vi "ethernet bc read.vi"(8 "error in":errorcluster, 11 "TCP Network Connection in":refnum<k5>) -> (2 "String":string, 3 "connection ID out":refnum<k5>)   [LabVIEW 2018]
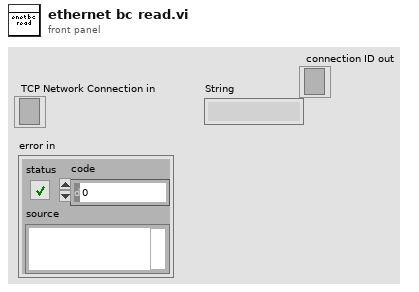
[diagram p1: front panel]
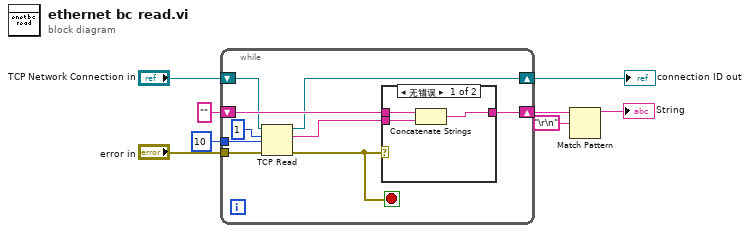
[diagram p0: block diagram]
diagram:
  n1 = while {
    tunnel: "error in" -> [w17]
    shift-right: [w14] -> w7
    shift-left: "" -> [w13]
    tunnel: 10 ("timeout ms (25000)") -> [w12]
    shift-right: [w9] -> w1
    shift-left: "TCP Network Connection in" -> [w10]
    stop <- w11 stop-if-true
    n2 = TCP Read(connection ID=w10, bytes to read=1, error in (no error)=w17, 9:w12) -> (connection ID out=w9:refnum<k5>, data out=w15:string, error out=w11:errorcluster)  [unwired: 1 in]
    n3 = case shown="无错误" w11 {
      tunnel: w15 -> [w19 _]
      tunnel: [w18 w21] -> w14
      tunnel: w13 -> [w20 w21]
      frame No Error {
        n4 = Concatenate Strings(w20, w19) -> (w18:string)
      }
      frame Error {
      }
    }
  }
  "connection ID out" <- w1
  n5 = Match Pattern(string=w7, regular expression="\r\n") -> (before substring=→"String":string)  [unwired: 1 in, 3 out]
